vi "Query Status.vi"(8 "error in (no error)":errorcluster, 9 "Mask Value(0)":dbl format="%#.2f", 10 "Command (0:*CLS)":u16(ring) items=["*CLS", "*ESE", "*ESE?", "*RST", "*SRE", "*SRE?", "*STB?", "*ESR?", "*IDN?", "*OPC", "*OPC?", "*TRG", "Output State", "Output-Timer", "Output-Timer-State"], 11 "VISA resource name":refnum<visa-resource-name>) -> (0 "error out":errorcluster, 2 "Instrument Response":string, 3 "VISA resource name out":refnum<visa-resource-name>)   [LabVIEW 2018, in "Keithley KE22xx Series.lvlib"]
doc: "Sends IEEE 488 common commands and returns the response for queries ."
uses:
  Keithley KE22xx Series.lvlib
panel:
  # "© 2012 Keithley Instruments, Inc. ALL RIGHTS RESERVED"
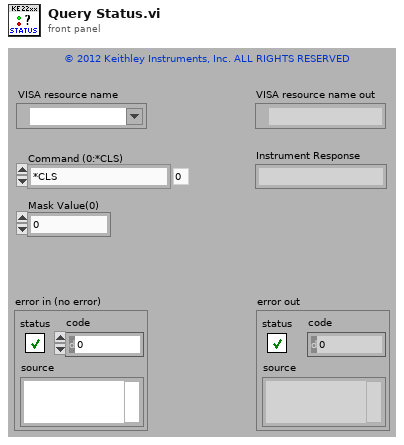
[diagram p1: front panel]
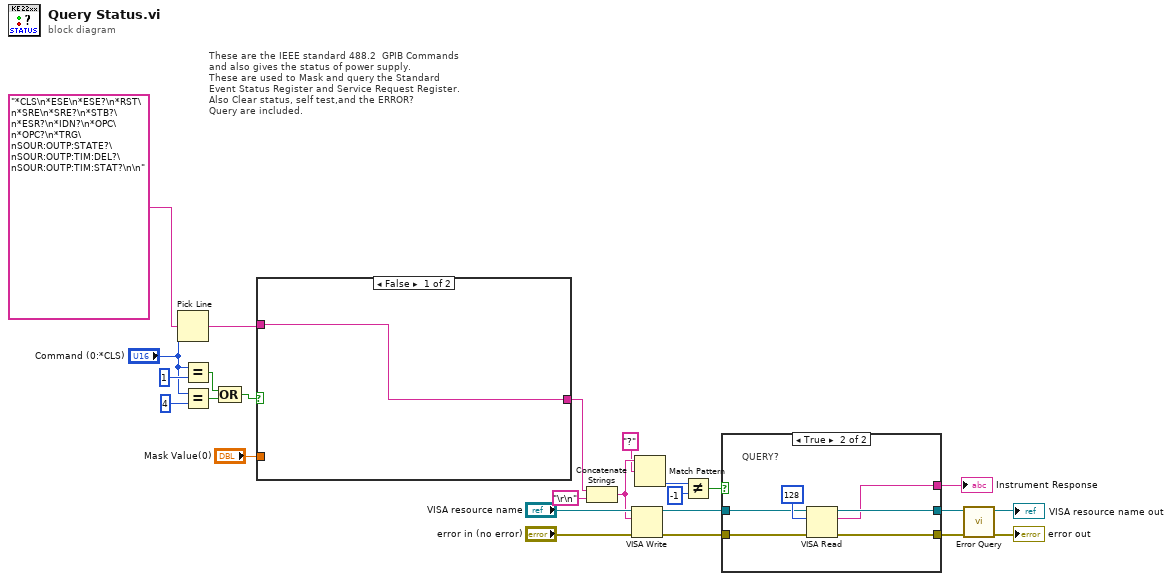
[diagram p0: block diagram]
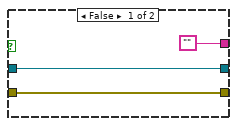
[diagram p2: hidden frame]
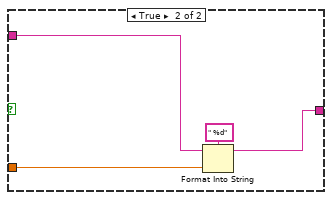
[diagram p3: hidden frame]
diagram:
  # "These are the IEEE standard 488.2  GPIB Commands\nand also gives the status of power supply.\nThese are used to Mask and query the Standard \nEvent Status Register and Service Request Register.  \nAlso Clear status, self test,and the ERROR?\nQuery are included."
  n1 = Pick Line(multi-line string="*CLS\n*ESE\n*ESE?\n*RST\n*SRE\n*SRE?\n*STB?\n*ESR?\n*IDN?\n*OPC\n*OPC?\n*TRG\nSOUR:OUTP:STATE?\nSOUR:OUTP:TIM:DEL?\nSOUR:OUTP:TIM:STAT?\n\n", line index="Command (0:*CLS)") -> (output string=w22:string)  [unwired: 1 out]
  n2 = Equal?(x="Command (0:*CLS)", y=u16 1) -> (x = y?=w21:bool)
  n3 = Equal?(x="Command (0:*CLS)", y=u16 4) -> (x = y?=w20:bool)
  n4 = Compound Arithmetic op=OR(w21, w20) -> (w17:bool)
  n5 = case shown="False" w17 {
    tunnel: w22 -> [w26 w29]
    tunnel: [w26 w28] -> w9
    tunnel: "Mask Value(0)" -> [_ w27]
    frame False {
    }
    frame True {
      n6 = Format Into String(format string=" %d", initial string=w29, w27) -> (resulting string=w28:string)  [unwired: 1 in, 1 out]
    }
  }
  n7 = Concatenate Strings(w9, "\r\n") -> (w8:string)
  n8 = VISA Write(VISA resource name="VISA resource name", write buffer=w8, error in (no error)="error in (no error)") -> (VISA resource name out=w14:refnum<visa-resource-name>, error out=w16:errorcluster)  [unwired: 1 out]
  n9 = Match Pattern(string=w8, regular expression="?") -> (offset past match=w23:i32)  [unwired: 4 out]
  n10 = Not Equal?(x=w23, y=-1) -> (x != y?=w15:bool)
  n11 = case shown="True" w15 {
    tunnel: [w33 w39] -> w4
    tunnel: w16 -> [w33 w38]
    tunnel: w14 -> [w32 w36]
    tunnel: [w32 w35] -> w5
    tunnel: ["" ("read buffer") w34] -> w10
    frame False {
    }
    frame True {
      # "QUERY?"
      n12 = VISA Read(VISA resource name=w36, byte count=u32 128, error in (no error)=w38) -> (VISA resource name out=w35:refnum<visa-resource-name>, read buffer=w34:string, error out=w39:errorcluster)  [unwired: 1 out]
    }
  }
  "Instrument Response" <- w10
  n13 = call "Error Query.vi"("error in (no error)"=w4, "VISA resource name"=w5) -> ("error out"=→"error out":errorcluster, "VISA resource name out"=→"VISA resource name out":refnum<visa-resource-name>)  [unwired: 6 in, 2 out]
